vi "Get GUID.vi"(8 "error in (no error)":errorcluster, 11 "SMO":refnum<class "SMO.lvclass">) -> (0 "error out":errorcluster, 2 "GUID":string, 3 "SMO out":refnum<class "SMO.lvclass">)   [LabVIEW 2021, in "smo.lvlib" / "SMO.lvclass"]
uses:
  SMO.lvclass
  Support/Attribute.Identity/Attribute.Identity.lvclass
  SMO.lvclass/SMO.ctl
  Support/Attribute.Identity/Attribute.Identity.lvclass/Attribute.Identity.ctl
  Private/ReftoDVR--SMO.vi
panel:
  # "This method is deprecated but kept for\nbackward-compatibility.\nUse the \"GetGUID.vi\" method instead of \"Get GUID.vi\""
  # "For instructions on how to use the JKI State Machine Objects, examples and video tutorials, visit:\nhttp://jki.net/state-machine-objects/\n\nJKI State Machine Objects™\nhttp://jki.net/state-machine-objects/\nCopyright (C) 2005-2015, JKI <info@jki.net>\nALL RIGHTS RESERVED"
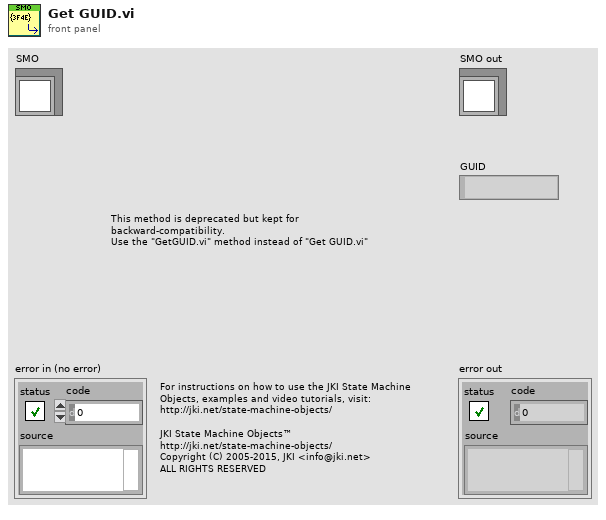
[diagram p1: front panel]
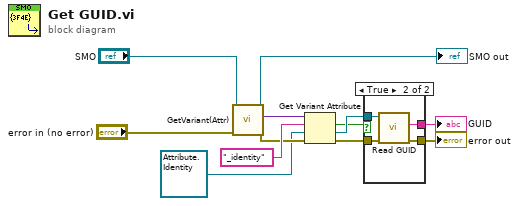
[diagram p0: block diagram]
diagram:
  n1 = call "GetVariant(Attr).vi"("error in (no error)"="error in (no error)", "SMO in"="SMO") -> ("error out"=w10:errorcluster, "[Attributes]"=w12:variant, "SMO out"=→"SMO out":refnum<class "SMO.lvclass">)  [unwired: 7 in]
  n2 = Get Variant Attribute(Variant=w12, name="_identity", default value (empty Variant)=refnum<class "Attribute.Identity.lvclass"> refnum, error in=w10) -> (found=w1:bool, value=w7:refnum<class "Attribute.Identity.lvclass">, error out=w8:errorcluster)  [unwired: 1 out]
  n3 = case shown="True" w1 {
    tunnel: w8 -> [w13 w17]
    tunnel: w7 -> [_ w16]
    tunnel: [_ w15] -> w3
    tunnel: [w13 w14] -> w2
    frame False {
    }
    frame True {
      n4 = call "Read GUID.vi"("error in (no error)"=w17, "Attribute.Identity in"=w16) -> ("error out"=w14:errorcluster, "GUID"=w15:string)  [unwired: 7 in, 1 out]
    }
  }
  "error out" <- w2
  "GUID" <- w3
